vi "cosine law.vi"() -> ()   [LabVIEW 2024]
panel:
  in  "angle":dbl
  in  "L2":dbl
  out "L_kr":dbl
  in  "L1":dbl
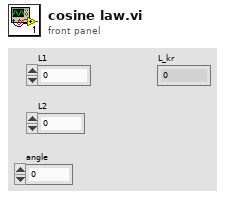
[diagram p1: front panel]
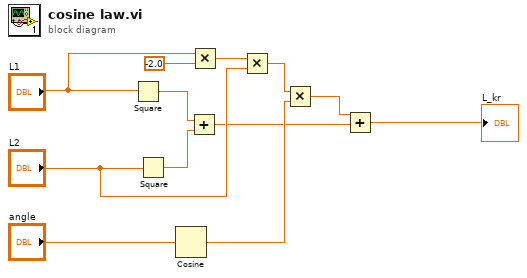
[diagram p0: block diagram]
diagram:
  n1 = Square(x="L1") -> (x^2=w12:dbl)
  n2 = Square(x="L2") -> (x^2=w5:dbl)
  n3 = Cosine(x="angle") -> (cos(x)=w6:dbl)
  n4 = Add(x=w12, y=w5) -> (x+y=w3:dbl)
  n5 = Multiply(x="L1", y=-2.0) -> (x*y=w9:dbl)
  n6 = Multiply(x=w9, y="L2") -> (x*y=w7:dbl)
  n7 = Multiply(x=w7, y=w6) -> (x*y=w2:dbl)
  n8 = Add(x=w2, y=w3) -> (x+y=→"L_kr":dbl)
